vi "solar_write VoyagerRefnum.vi"(8 "error in (no error)":errorcluster, 10 "VoyagerRefnum":T1, 11 "solar in":refnum<class "solar.lvclass">) -> (0 "error out":errorcluster, 3 "solar out":refnum<class "solar.lvclass">)   [LabVIEW 2018, in "solar.lvclass"]
doc: "Writes a new Voyager Refnum to the SOLAR object."
uses:
  solar.lvclass
  voyager/solar_voy_ctl Voyager Refnum.ctl
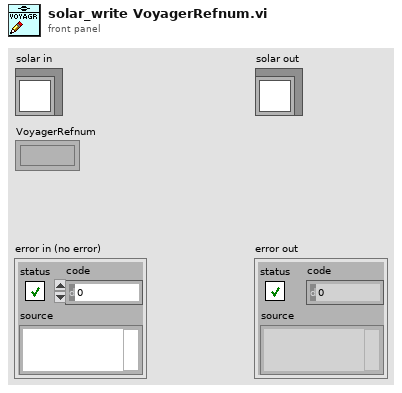
[diagram p1: front panel]
types:
  T1 = typedef "solar_voy_ctl Voyager Refnum.ctl" = refnum<k1>
  T2 = typedef "solar_ctl SOLAR Refnum.ctl" = refnum<k1>
  T3 = typedef "solar_ctl SOLAR Global.ctl" = cluster{"Targets":T4[], "AppDir":path, "solar.ini":path, "ConfigsDir":path, "CosmosDir":path, "LogsDir":path, "ExePath":path, "ExeVersion":string, "PartNum":string, "AppSetup":string, "Title":string, "Main.ini":path, "Temp.ini":path, "vSOLAR":string, "Splash.png":string, "SplashWait":i32, "SOLARUE":refnum<user-event>, "VoyagerRefnum":T1, "QTimerRefnum":T5}
  T4 = typedef "solar_ctl Target Global.ctl" = cluster{"Target":string, "Q":refnum<queue>, "UE":refnum<user-event>, "VI":refnum<vi>, "Menu":refnum<k9>, "Data":refnum<data-value>, "Attributes":variant}
  T5 = typedef "solar_qtimer_ctl Refnum.ctl" = refnum<k1>
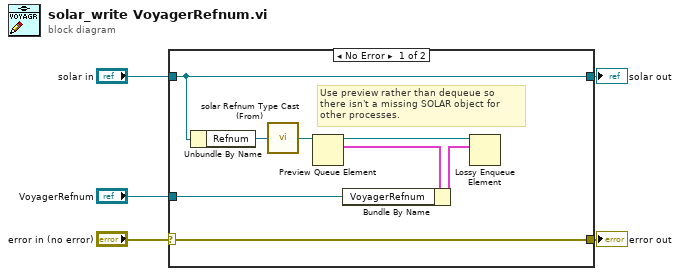
[diagram p0: block diagram]
diagram:
  n1 = case shown="No Error" "error in (no error)" {
    selector: "error in (no error)" -> [w13 w15]
    tunnel: "solar in" -> [w11 w14]
    tunnel: [w13 w15] -> w3
    tunnel: [w11 w14] -> w4
    tunnel: "VoyagerRefnum" -> [w7 _]
    frame No Error {
      # "Use preview rather than dequeue so there isn't a missing SOLAR object for other processes."
      n2 = Unbundle By Name(w11) -> ("Refnum"=w10:T2)
      n3 = call "solar Refnum Type Cast (From).vi"("Refnum"=w10) -> ("SOLAR"=w12:refnum<queue>)
      n4 = Preview Queue Element(queue=w12) -> (queue out=w8:refnum<queue>, element=w9:T3)  [unwired: 2 in, 2 out]
      n5 = Bundle By Name(cluster=w9, "VoyagerRefnum"=w7) -> (w6:T3)
      n6 = Lossy Enqueue Element(queue=w8, element=w6) -> ()  [unwired: 1 in, 4 out]
    }
    frame Error {
    }
  }
  "error out" <- w3
  "solar out" <- w4
